vi "Read Gear Wings V.5.0.vi"(11 "Joystick Buttons":bool[](array[boolean])) -> ()   [LabVIEW 2016]
uses:
  Robot Global Data V.5.0.vi
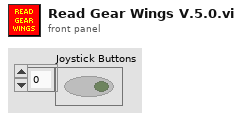
[diagram p1: front panel]
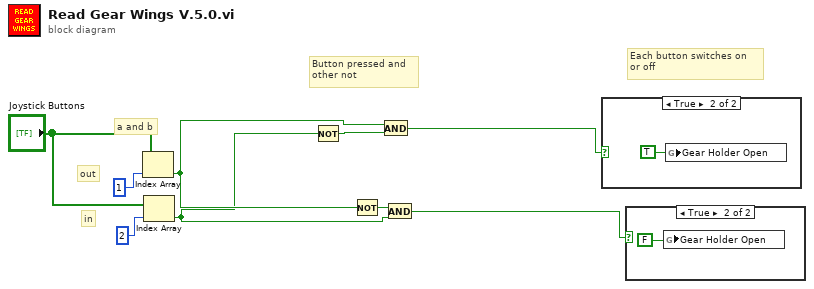
[diagram p0: block diagram]
diagram:
  # "Button pressed and \nother not"
  # "Each button switches on \nor off"
  # "a and b"
  # "in"
  # "out"
  n1 = Index Array(array="Joystick Buttons", index=1) -> (element=w4:bool)
  n2 = Index Array(array="Joystick Buttons", index=2) -> (element=w3:bool)
  n3 = Not(x=w3) -> (.not. x?=w7:bool)
  n4 = Not(x=w4) -> (.not. x?=w6:bool)
  n5 = And(x=w4, y=w7) -> (x .and. y?=w2:bool)
  n6 = And(x=w6, y=w3) -> (x .and. y?=w5:bool)
  n7 = case shown="True" w2 {
    frame False {
    }
    frame True {
      n8 = global write "Robot Global Data V.5.0.vi" "Gear Holder Open"(TRUE) -> ()
    }
  }
  n9 = case shown="True" w5 {
    frame False {
    }
    frame True {
      n10 = global write "Robot Global Data V.5.0.vi" "Gear Holder Open"(FALSE) -> ()
    }
  }
